vi "tutorial ex.vi"() -> ()   [LabVIEW 2011]
uses:
  <vilib>/Utility/file.llb/Read From Spreadsheet File (string).vi
panel:
  out "text":string
  out "all rows":string[][](array[string])
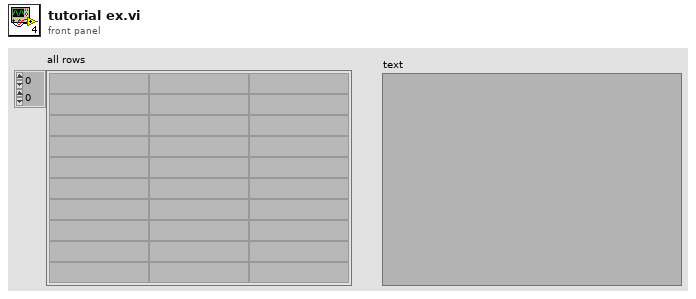
[diagram p1: front panel]
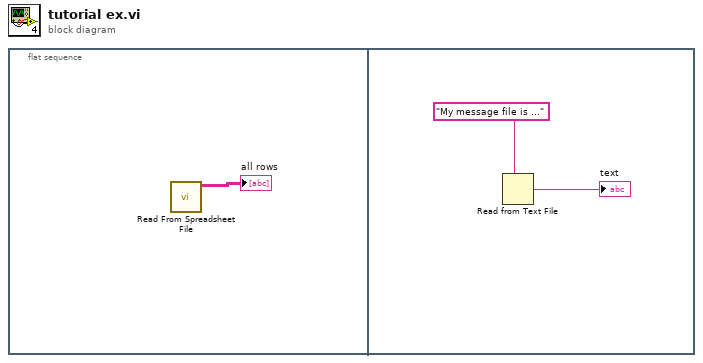
[diagram p0: block diagram]
diagram:
  n1 = flat-sequence {
    frame #0 {
      n2 = call-poly <vilib>:"Read From Spreadsheet File.vi"() -> ("all rows"=→"all rows":string[][])  [unwired: 7 in, 4 out]
    }
    frame #1 {
      n3 = Read from Text File(prompt (Open existing file)="My message file is ...") -> (text=→"text":string)  [unwired: 3 in, 3 out]
    }
  }
